vi "Write Byte.vi"(7 "Mode (Command)":T1, 8 "error in (no error)":errorcluster, 9 "Value":u8 format="%.0x", 11 "PCF8574 I2C LCD in":refnum<class "PCF8574 I2C LCD.lvclass">) -> (0 "error out":errorcluster, 3 "PCF8574 I2C LCD out":refnum<class "PCF8574 I2C LCD.lvclass">)   [LabVIEW 2020, in "CTI-Peripheral.lvlib" / "PCF8574 I2C LCD.lvclass"]
uses:
  PCF8574 I2C LCD.lvclass
  Mode.ctl
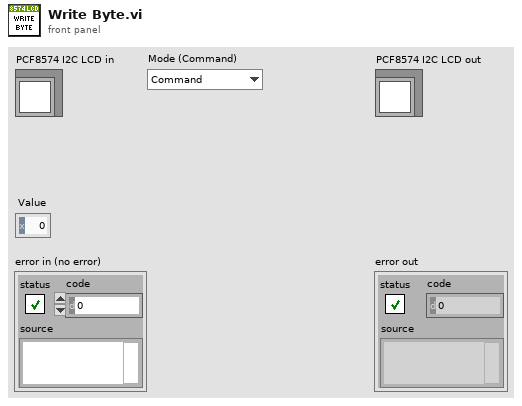
[diagram p1: front panel]
types:
  T1 = typedef "CTI-Peripheral.lvlib/PCF8574 I2C LCD.lvclass/Mode.ctl" = enum8{"Command", "Character"}
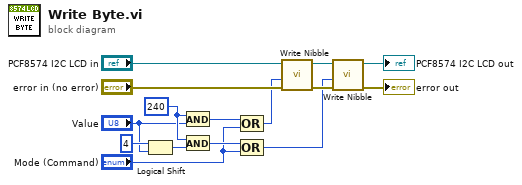
[diagram p0: block diagram]
diagram:
  w12 = u8 240 ("y")
  n1 = Logical Shift(y=i16 4, x="Value") -> (x << y=w13:u8)
  n2 = And(x=w12, y="Value") -> (x .and. y?=w11:u8)
  n3 = And(x=w12, y=w13) -> (x .and. y?=w10:u8)
  n4 = Compound Arithmetic op=OR(w11, "Mode (Command)") -> (w6:u8)
  n5 = Compound Arithmetic op=OR(w10, "Mode (Command)") -> (w3:u8)
  n6 = call "Write Nibble.vi"("error in (no error)"="error in (no error)", "Value"=w6, "PCF8574 I2C LCD in"="PCF8574 I2C LCD in") -> ("error out"=w4:errorcluster, "PCF8574 I2C LCD out"=w5:refnum<class "PCF8574 I2C LCD.lvclass">)  [unwired: 7 in]
  n7 = call "Write Nibble.vi"("error in (no error)"=w4, "Value"=w3, "PCF8574 I2C LCD in"=w5) -> ("error out"=→"error out":errorcluster, "PCF8574 I2C LCD out"=→"PCF8574 I2C LCD out":refnum<class "PCF8574 I2C LCD.lvclass">)  [unwired: 7 in]
